vi "AWS_Retrieve_IoT_Data.vi"() -> ()   [LabVIEW 2017]
uses:
  <vilib>/AWS Toolkit/IoT/IoT Session/IoT Session.lvclass
  <vilib>/AWS Toolkit/IoT/Thing Shadow/Thing Shadow.lvclass
  <vilib>/AWS Toolkit/Core/HTTP Request/AWS Credentials.ctl
  <vilib>/AWS Toolkit/Core/HTTP Request/HTTP Request.lvclass
  <vilib>/AWS Toolkit/Core/HTTP Request/Region.ctl
panel:
  in  "Region":T1
  in  "AWS Credentials":T2
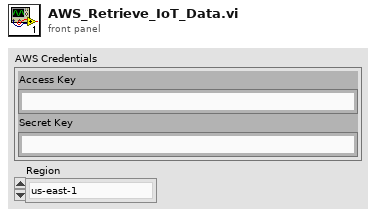
[diagram p1: front panel]
types:
  T1 = typedef "NI_AWS_Core.lvlib/HTTP Request.lvclass/Region.ctl" = enum16{"us-east-1", "us-east-2", "us-west-1", "us-west-2", "ap-northeast-1", "ap-northeast-2", "ap-southeast-1", "ap-southeast-2", "ca-central-1", "eu-central-1", "eu-west-1", "eu-west-2", "sa-east-1"}
  T2 = typedef "NI_AWS_Core.lvlib/HTTP Request.lvclass/AWS Credentials.ctl" = cluster{"Access Key":string, "Secret Key":string}
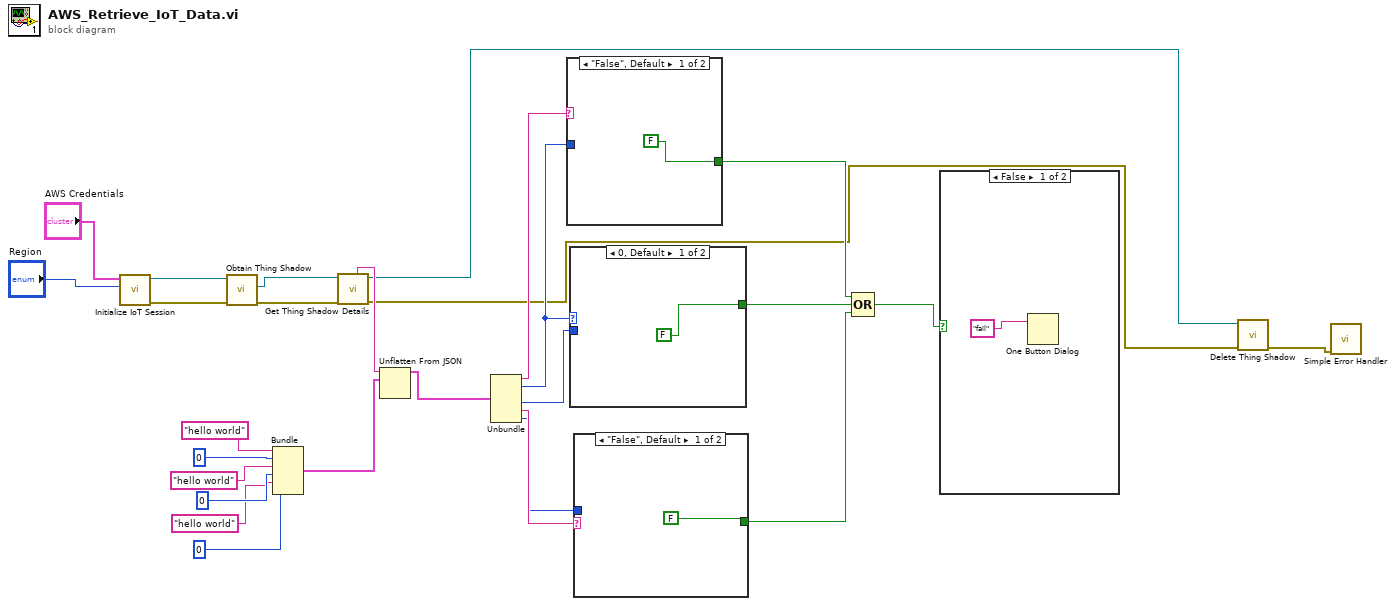
[diagram p0: block diagram]
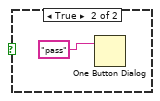
[diagram p2: hidden frame]
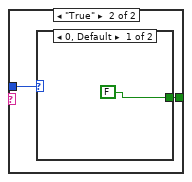
[diagram p3: hidden frame]
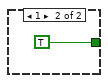
[diagram p4: hidden frame]
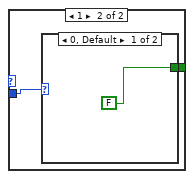
[diagram p5: hidden frame]
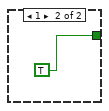
[diagram p6: hidden frame]
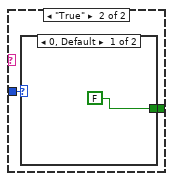
[diagram p7: hidden frame]
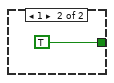
[diagram p8: hidden frame]
diagram:
  n1 = call <vilib>:"Initialize IoT Session.vi"("Region"="Region", "AWS Credentials"="AWS Credentials") -> ("error out"=w24:errorcluster, "IoT Session"=w27:refnum<class "IoT Session.lvclass">)  [unwired: 8 in]
  n2 = call <vilib>:"Obtain Thing Shadow.vi"("error in (no error)"=w24, "IoT Session in"=w27) -> ("error out"=w4:errorcluster, "Shadow Thing"=w23:refnum<class "Thing Shadow.lvclass">)  [unwired: 7 in, 1 out]
  n3 = Bundle("hello world", 0, "hello world", 0, "hello world", 0) -> (w20:cluster{string, i32, string, i32, string, i32})  [unwired: 1 in]
  n4 = call <vilib>:"Get Thing Shadow Details.vi"("error in (no error)"=w4, "Thing Shadow in"=w23) -> ("error out"=w1:errorcluster, "Thing Shadow out"=w3:refnum<class "Thing Shadow.lvclass">, "Raw JSON"=w19:string)  [unwired: 4 in, 3 out]
  n5 = Unflatten From JSON(JSON string=w19, type and defaults=w20) -> (value=w18:cluster{string, i32, string, i32, string, i32})  [unwired: 5 in, 1 out]
  n6 = Unbundle(w18) -> (w13:string, w12:i32, w11:i32, w10:string, w9:i32)  [unwired: 1 out]
  n7 = case shown="\"False\", Default" w13 {
    tunnel: w12 -> [_ w30]
    tunnel: [FALSE w29] -> w6
    frame "False", Default {
    }
    frame "True" {
      n8 = case shown="0, Default" w30 {
        tunnel: [FALSE TRUE] -> w29
        frame 0, Default {
        }
        frame 1 {
        }
      }
    }
  }
  n9 = case shown="0, Default" w12 {
    tunnel: w11 -> [_ w35]
    tunnel: [FALSE w34] -> w7
    frame 0, Default {
    }
    frame 1 {
      n10 = case shown="0, Default" w35 {
        tunnel: [FALSE TRUE] -> w34
        frame 0, Default {
        }
        frame 1 {
        }
      }
    }
  }
  n11 = case shown="\"False\", Default" w10 {
    tunnel: w9 -> [_ w40]
    tunnel: [FALSE w39] -> w8
    frame "False", Default {
    }
    frame "True" {
      n12 = case shown="0, Default" w40 {
        tunnel: [FALSE TRUE] -> w39
        frame 0, Default {
        }
        frame 1 {
        }
      }
    }
  }
  n13 = Compound Arithmetic op=OR(w6, w7, w8) -> (w5:bool)
  n14 = case shown="False" w5 {
    frame False {
      n15 = One Button Dialog(message="fail") -> ()  [unwired: 1 in, 1 out]
    }
    frame True {
      n16 = One Button Dialog(message="pass") -> ()  [unwired: 1 in, 1 out]
    }
  }
  n17 = call <vilib>:"Delete Thing Shadow.vi"("error in (no error)"=w1, "Thing Shadow"=w3) -> ("error out"=w2:errorcluster)  [unwired: 9 in]
  n18 = call <vilib>:"Simple Error Handler.vi"("error in (no error)"=w2) -> ()  [unwired: 4 in, 5 out]
